vi "main_save_projector_images.vi"(8 "error in":errorcluster, 10 "Array":T1[](array[typedef]), 11 "Queue in":refnum<queue>) -> (0 "error out":errorcluster)   [LabVIEW 2019]
uses:
  <vilib>/vision/Image Controls.llb/IMAQ Image.ctl
  ParametersGlobal.vi
  DebugGlobal.vi
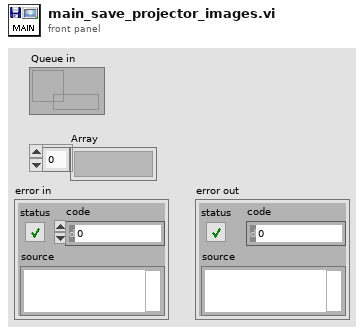
[diagram p1: front panel]
types:
  T1 = typedef "IMAQ Image.ctl" = refnum<image>
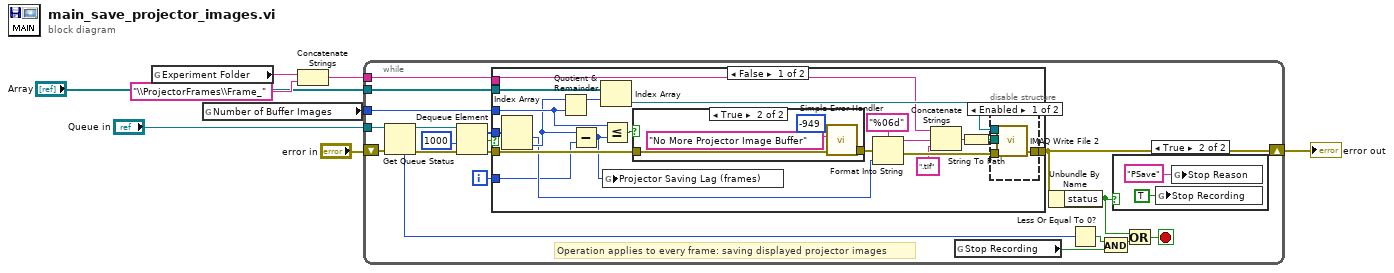
[diagram p0: block diagram]
diagram:
  n1 = global read "ParametersGlobal.vi" "Experiment Folder"() -> (w5:string)
  n2 = global read "ParametersGlobal.vi" "Number of Buffer Images"() -> (w8:i32)
  n3 = Concatenate Strings(w5, "\\ProjectorFrames\\Frame_" ("string")) -> (w7:string)
  n4 = while {
    shift-right: [w17] -> w2
    shift-left: "error in" -> [w25]
    tunnel: "Queue in" -> [w26]
    tunnel: "Array" -> [w21]
    tunnel: w8 -> [w20]
    tunnel: w7 -> [w16]
    i -> [w13]
    stop <- w22 stop-if-true
    # "Operation applies to every frame: saving displayed projector images"
    n5 = Get Queue Status(queue=w26, error in (no error)=w25) -> (queue out=w27:refnum<queue>, error out=w24:errorcluster, # elements in queue=w10:i32)  [unwired: 1 in, 5 out]
    n6 = Dequeue Element(queue=w27, timeout in ms (-1)=1000, error in (no error)=w24) -> (element=w18:i32[], timed out?=w14:bool, error out=w19:errorcluster)  [unwired: 1 out]
    n7 = case shown="False" w14 {
      tunnel: w21 -> [w48 _]
      tunnel: w20 -> [w47 _]
      tunnel: w19 -> [w46 w60]
      tunnel: w18 -> [w44 _]
      tunnel: [w36 w60] -> w17
      tunnel: w16 -> [w33 _]
      tunnel: w13 -> [w31 _]
      frame False {
        n8 = Index Array(array=w44) -> (element #1=w40:i32, element #2=w43:i32)  [unwired: 2 in]
        n9 = Quotient & Remainder(x=w43, y=w47) -> (x-y*floor(x/y)=w49:i32)  [unwired: 1 out]
        n10 = Subtract(x=w43, y=w31) -> (x-y=w30:i32)
        n11 = Index Array(array=w48, index=w49) -> (element=w35:T1)
        n12 = Less Or Equal?(x=w47, y=w30) -> (x <= y?=w45:bool)
        n13 = global write "DebugGlobal.vi" "Projector Saving Lag (frames)"(w30) -> ()
        n14 = case shown="True" w45 {
          tunnel: w46 -> [w55 w59]
          tunnel: [w55 w58] -> w41
          frame False {
          }
          frame True {
            n15 = call <vilib>:"Simple Error Handler.vi"("error code (no error:0)"=-949, "error source (\" \")"="No More Projector Image Buffer" ("error source (\" \")"), "error in (no error)"=w59) -> ("error out"=w58:errorcluster)  [unwired: 2 in, 4 out]
          }
        }
        n16 = Format Into String(format string="%06d" ("string"), error in=w41, w40) -> (resulting string=w34:string, error out=w37:errorcluster)  [unwired: 1 in]
        n17 = Concatenate Strings(w33, w34, ".tif" ("string")) -> (w39:string)
        n18 = String To Path(string=w39) -> (path=w38:path)
        n19 = disable-structure shown="Enabled" {
          disable-tunnel: w38 -> [w53 _]
          disable-tunnel: w37 -> [w52 w54]
          disable-tunnel: [w51 w54] -> w36
          disable-tunnel: w35 -> [w50 _]
          frame Enabled {
            n20 = call-poly "IMAQ Write File 2"("error in (no error)"=w52, "File Path"=w53, "Image"=w50) -> ("error out"=w51:errorcluster)  [unwired: 7 in, 1 out]
          }
          frame Disabled {
          }
        }
      }
      frame True {
      }
    }
    n21 = global read "DebugGlobal.vi" "Stop Recording"() -> (w12:bool)
    n22 = Unbundle By Name(w17) -> ("status"=w11:bool)
    n23 = Less Or Equal To 0?(x=w10) -> (x <= 0?=w9:bool)
    n24 = And(x=w9, y=w12) -> (x .and. y?=w23:bool)
    n25 = case shown="True" w11 {
      frame False {
      }
      frame True {
        n26 = global write "DebugGlobal.vi" "Stop Recording"(TRUE ("stop")) -> ()
        n27 = global write "DebugGlobal.vi" "Stop Reason"("PSave" ("Stop Debug")) -> ()
      }
    }
    n28 = Or(x=w11, y=w23) -> (x .or. y?=w22:bool)
  }
  "error out" <- w2
